vi "Flankenauswertung_SPS.vi"(9 "SPS IN":T2, 11 "Schieberegister in":T2) -> (1 "Event out":T1, 2 "Positive Flanke":bool, 3 "Schieberegister out":T2)   [LabVIEW 2024]
doc: "Prüft ob die Eingangsvariablen von der SPS ihren Wert geändert haben und gibt den dazugehörigen Zustand, welcher gestartet werden soll aus."
uses:
  Typdefinitionen/Cluster_SPS_IN.ctl
  Typdefinitionen/Zustand.ctl
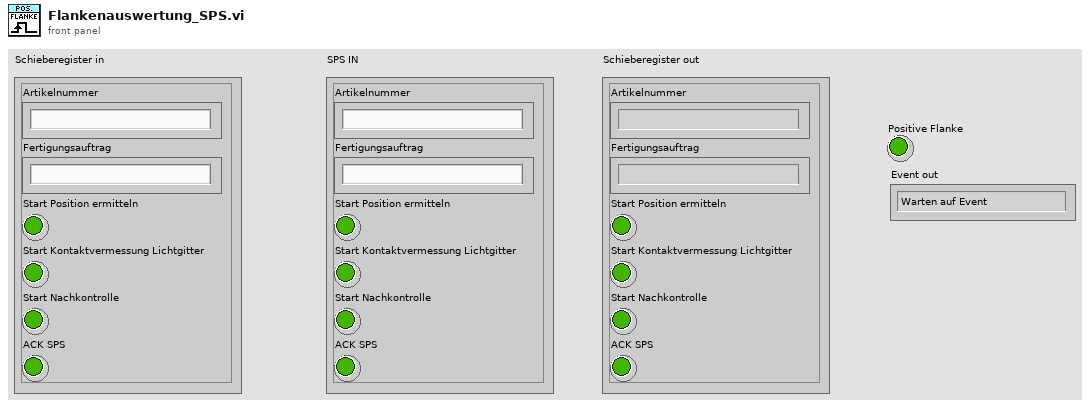
[diagram p1: front panel]
types:
  T1 = typedef "Zustand.ctl" = enum16{"Warten auf Event", "Artikeldaten laden", "Init Prüfung Oben", "Bildaufnahme Oben", "Auswertung Oben", "Bilder Oben speichern", "Init Vermessung Lichtgitter", "Messwertaufnahme Lichtgitter", "Auswertung Lichtgitter", "Init Prüfung Unten", "Bildaufnahme Unten", "Auswertung Unten", "Bild Unten speichern", "Fehler quittieren"}
  T2 = typedef "Cluster_SPS_IN.ctl" = cluster{"Artikelnummer":string, "Fertigungsauftrag":string, "Start Position ermitteln":bool, "Start Kontaktvermessung Lichtgitter":bool, "Start Nachkontrolle":bool, "ACK SPS":bool}
  T3 = cluster{"Artikelnummer":bool, "Fertigungsauftrag":bool, "Start Position ermitteln":bool, "Start Kontaktvermessung Lichtgitter":bool, "Start Nachkontrolle":bool, "ACK SPS":bool}
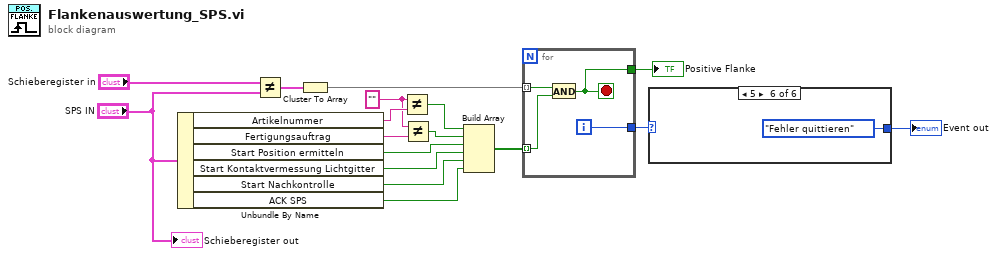
[diagram p0: block diagram]
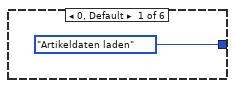
[diagram p2: hidden frame]
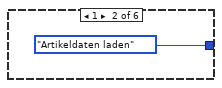
[diagram p3: hidden frame]
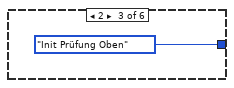
[diagram p4: hidden frame]
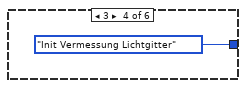
[diagram p5: hidden frame]
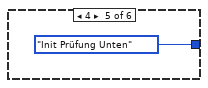
[diagram p6: hidden frame]
diagram:
  w3 = "" ("x")
  n1 = Unbundle By Name("SPS IN") -> ("Artikelnummer"=w4:string, "Fertigungsauftrag"=w5:string, "Start Position ermitteln"=w6:bool, "Start Kontaktvermessung Lichtgitter"=w12:bool, "Start Nachkontrolle"=w11:bool, "ACK SPS"=w1:bool)
  n2 = Not Equal?(x="Schieberegister in", y="SPS IN") -> (x != y?=w15:T3)
  n3 = Cluster To Array(cluster=w15) -> (array=w14:bool[])
  n4 = Not Equal?(x=w3, y=w4) -> (x != y?=w7:bool)
  n5 = Not Equal?(x=w3, y=w5) -> (x != y?=w2:bool)
  n6 = Build Array(w7, w2, w6, w12, w11, w1) -> (w10:bool[])
  n7 = for {
    tunnel: w14 -> [w21] mode=indexing
    tunnel: w10 -> [w20] mode=indexing
    tunnel: [w19] -> w9
    tunnel: [w18] -> w8
    i -> [w19]
    stop <- w18 stop-if-true
    n8 = And(x=w21, y=w20) -> (x .and. y?=w18:bool)
  }
  "Positive Flanke" <- w8
  n9 = case shown="5" w9 {
    tunnel: [Zustand."Artikeldaten laden" ("Enum") Zustand."Artikeldaten laden" ("Enum") Zustand."Init Prüfung Oben" ("Enum") Zustand."Init Vermessung Lichtgitter" ("Enum") Zustand."Init Prüfung Unten" ("Enum") Zustand."Fehler quittieren" ("Enum")] -> w17
    frame 0, Default {
    }
    frame 1 {
    }
    frame 2 {
    }
    frame 3 {
    }
    frame 4 {
    }
    frame 5 {
    }
  }
  "Event out" <- w17
  "Schieberegister out" <- "SPS IN"
